vi "hello VI.vi"() -> ()   [LabVIEW 2026]
panel:
  in  "INPUT 2":dbl
  out "OUTPUT":dbl
  in  "INPUT 1":dbl
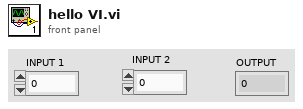
[diagram p1: front panel]
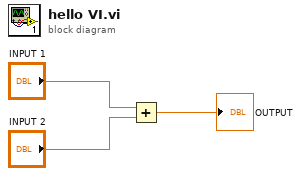
[diagram p0: block diagram]
diagram:
  n1 = Add(x="INPUT 1", y="INPUT 2") -> (x+y=→"OUTPUT":dbl)
